vi "Signal Constructor.vi"(8 "error in (no error)":errorcluster, 11 "Signal Settings":T1) -> (0 "error out":errorcluster, 3 "IO Class.lvclass":refnum<class "Signal.lvclass">)   [LabVIEW 2025, in "Signal.lvclass"]
uses:
  Signal.lvclass
  Signal Settings.ctl
  Configuration.ctl
  VI/VI/Error Codes.ctl
  Digital Indicator/Digital Indicator.lvclass
  C:/Projects/VeriStand-FPGA-Generation-Wizard/Source/Classes/Signal/Signal/Signal.lvclass
  Digital Control/Digital Control.lvclass
  Analog Indicator/Analog Indicator.lvclass
  Analog Control/Analog Control.lvclass
  FPGA Addon Input/FPGA Addon Input.lvclass
  FPGA Addon Output/FPGA Addon Output.lvclass
  Quadrature Encoder Input/Quadrature Encoder Input.lvclass
  Wheel Speed Sensor/Wheel Speed Sensor.lvclass
  Signal.lvclass/Signal.ctl
  EST Digital Event/Digital Event.lvclass
  EST Output/EST Output.lvclass
  EST Knock Sensor/Knock Sensor.lvclass
  VI/VI/VI.lvclass
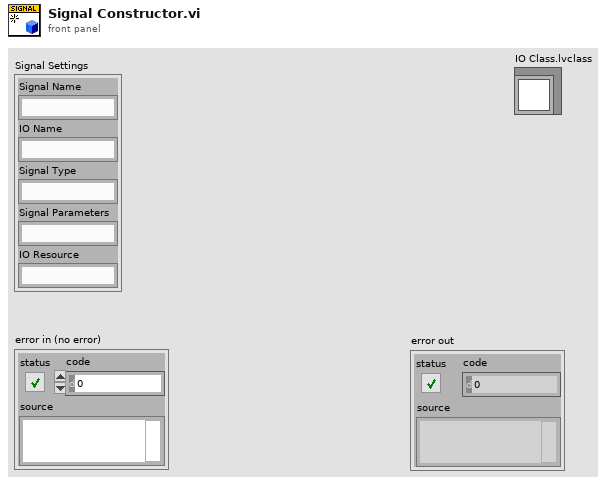
[diagram p1: front panel]
types:
  T1 = typedef "Signal.lvclass/Signal Settings.ctl" = cluster{"Signal Name":string, "IO Name":string, "Signal Type":string, "Signal Parameters":string, "IO Resource":string}
  T2 = typedef "VI.lvclass/Error Codes.ctl" = enum16{"Signal Unsupported", "Module Unsupported", "Parameter Unsupported", "Signal Code Gen Error", "Module Code Gen Error", "Cleanup Code Error", "Signal Direction Mismatch", "Signal Type Mismatch", "Module Channel Number Mismatch", "Minimum Channels Mismatch"}
  T3 = typedef "Signal.lvclass/Configuration.ctl" = cluster{"Classification":string, "Direction":string, "Type":string}
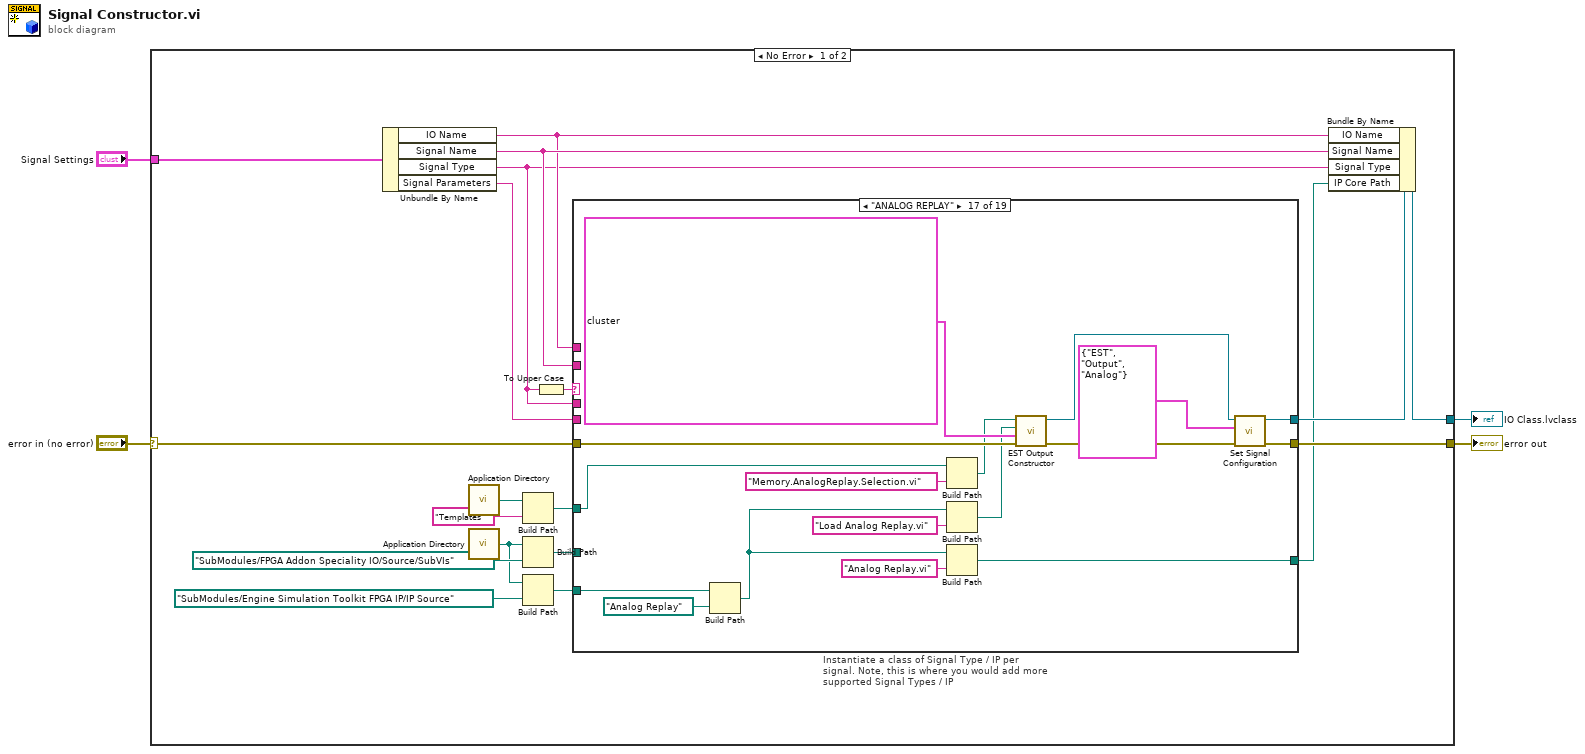
[diagram p0: block diagram]
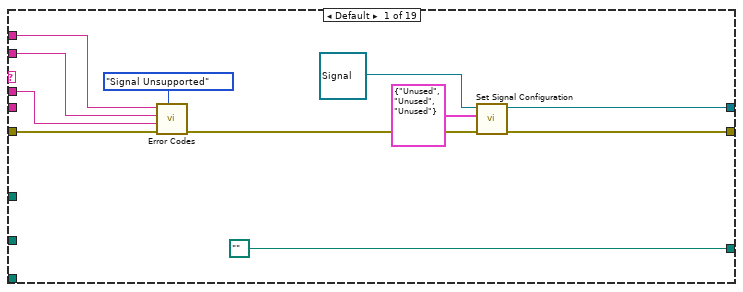
[diagram p2: hidden frame]
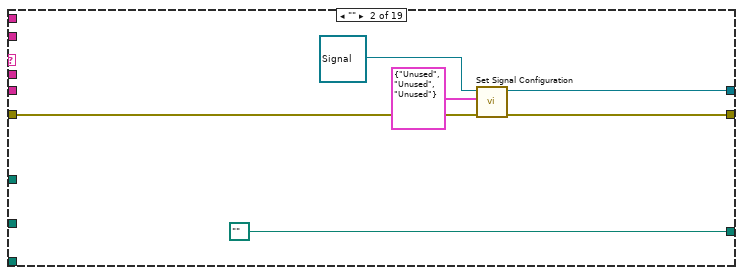
[diagram p3: hidden frame]
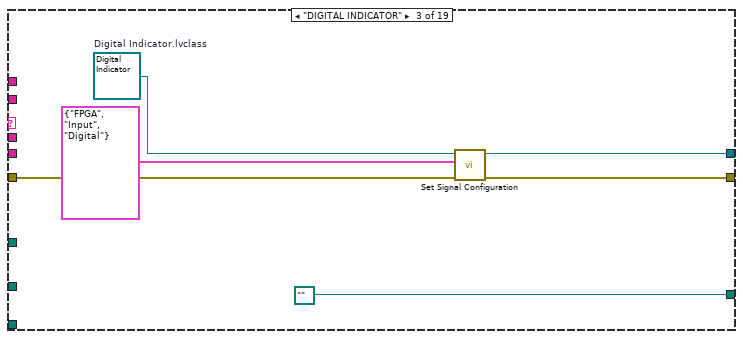
[diagram p4: hidden frame]
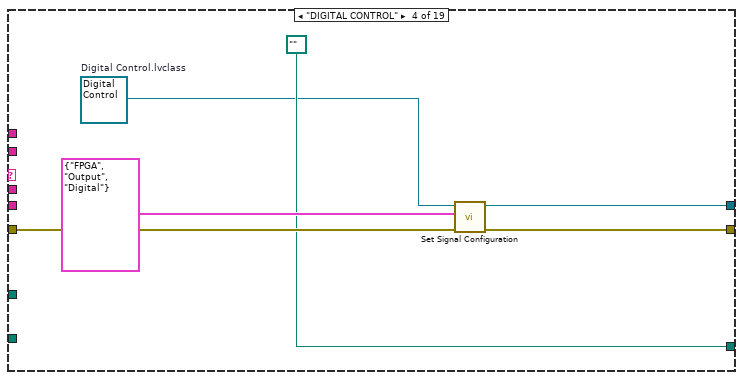
[diagram p5: hidden frame]
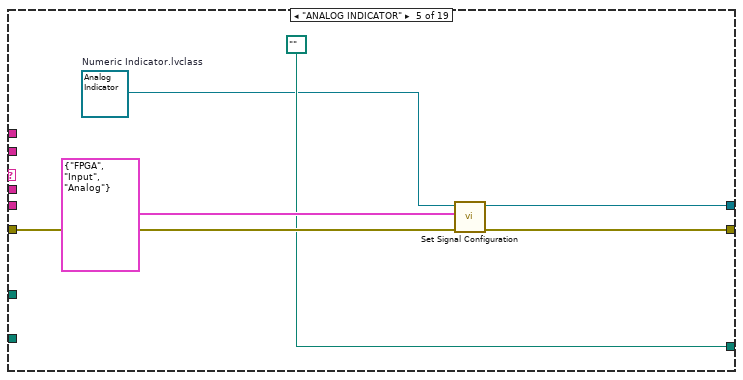
[diagram p6: hidden frame]
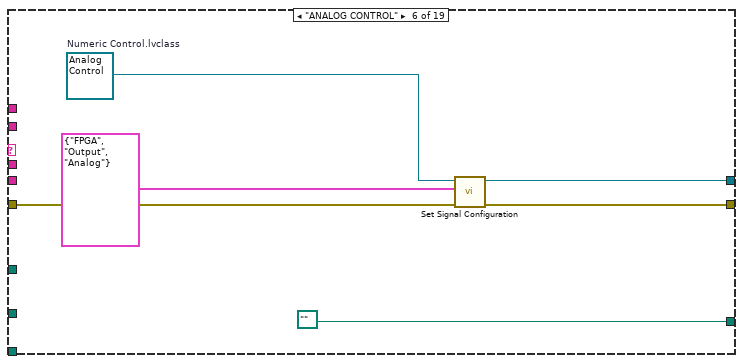
[diagram p7: hidden frame]
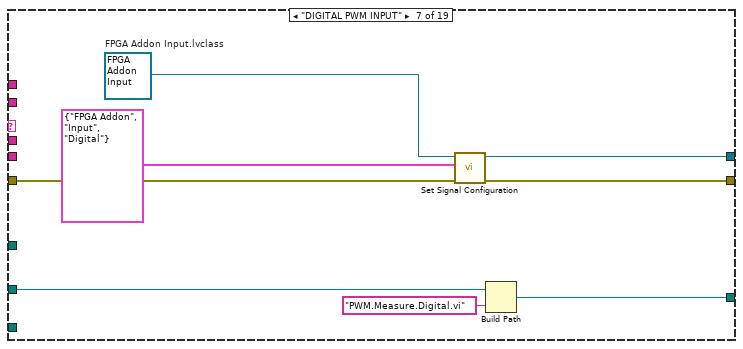
[diagram p8: hidden frame]
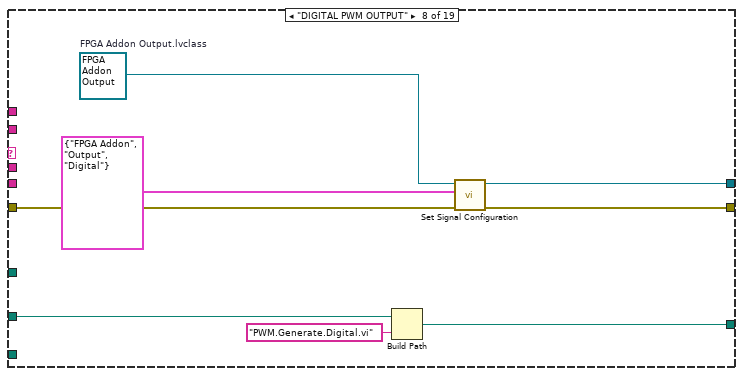
[diagram p9: hidden frame]
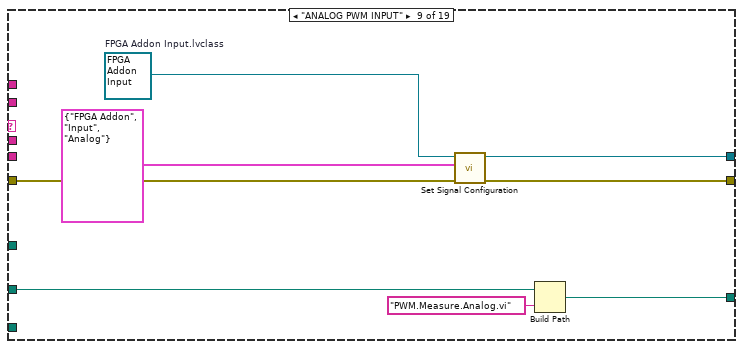
[diagram p10: hidden frame]
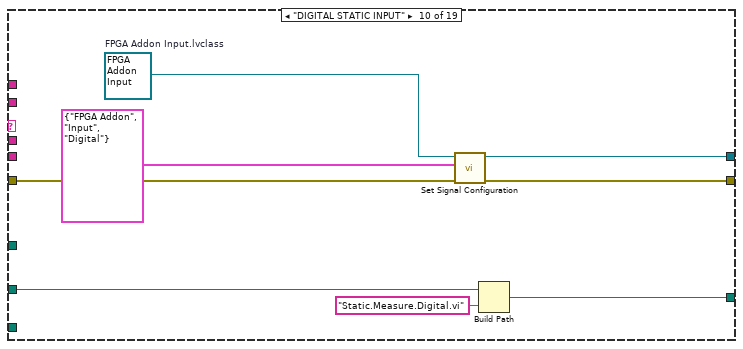
[diagram p11: hidden frame]
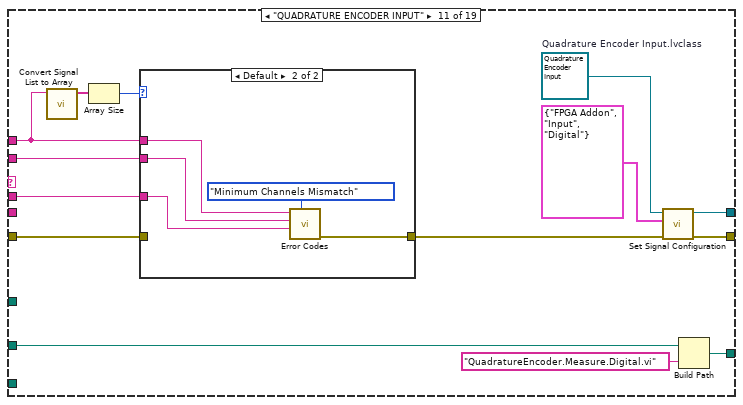
[diagram p12: hidden frame]
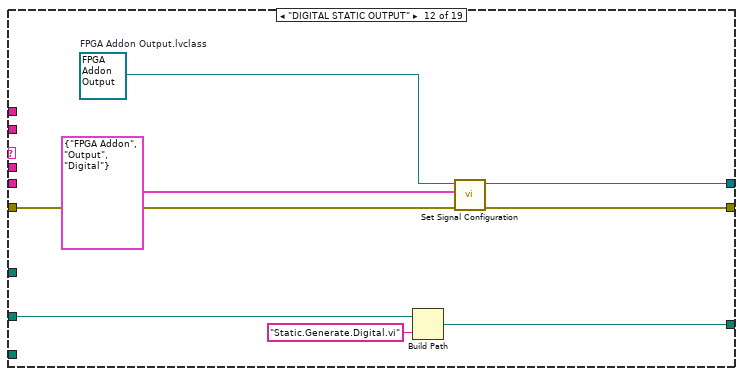
[diagram p14: hidden frame]
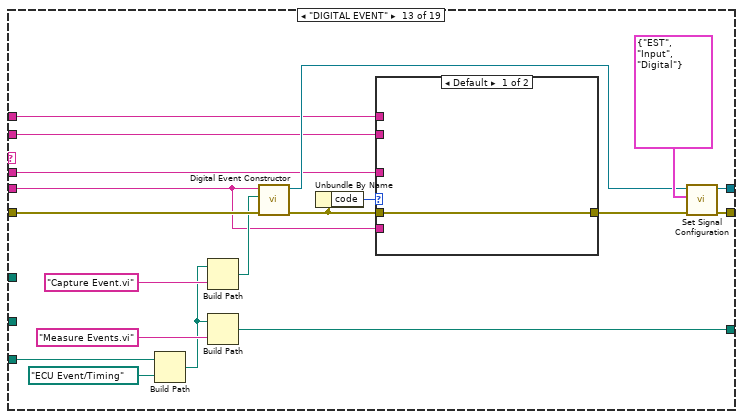
[diagram p15: hidden frame]
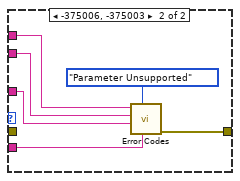
[diagram p16: hidden frame]
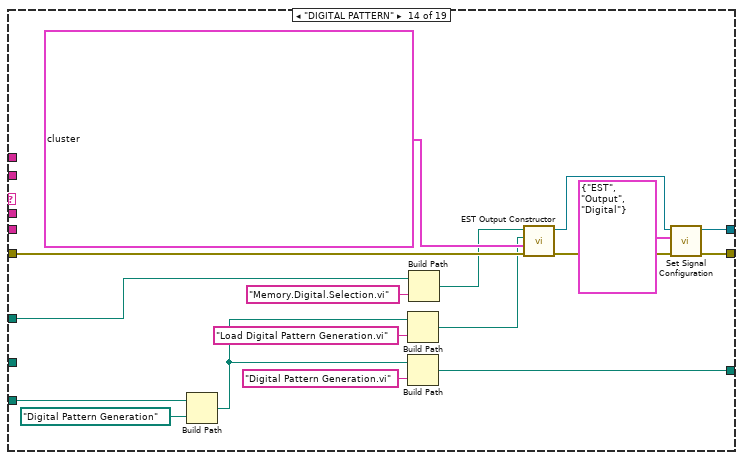
[diagram p17: hidden frame]
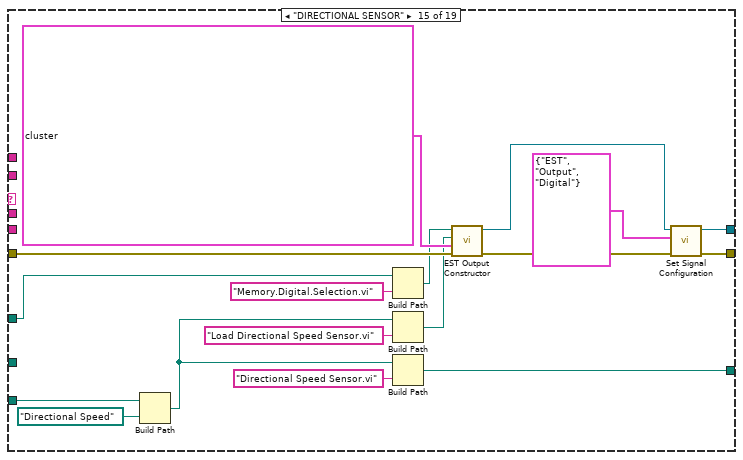
[diagram p18: hidden frame]
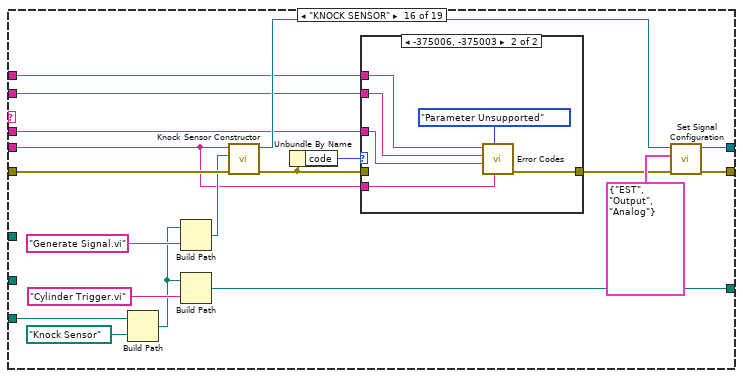
[diagram p19: hidden frame]
diagram:
  n1 = case shown="No Error" "error in (no error)" {
    selector: "error in (no error)" -> [w5 w257]
    tunnel: "Signal Settings" -> [w23 _]
    tunnel: [w21 w257] -> w3
    tunnel: [w20 refnum<class "Signal.lvclass"> refnum ("IO Class out")] -> w2
    frame No Error {
      n2 = Unbundle By Name(w23) -> ("IO Name"=w7:string, "Signal Name"=w8:string, "Signal Type"=w6:string, "Signal Parameters"=w19:string)
      n3 = call <vilib>:"Application Directory.vi"() -> ("Application Directory"=w11:path)
      n4 = call <vilib>:"Application Directory.vi"() -> ("Application Directory"=w9:path)
      n5 = Build Path(base path=w11, name or relative path="Templates") -> (appended path=w10:path)
      n6 = Build Path(base path=w9, name or relative path=path "SubModules/FPGA Addon Speciality IO/Source/SubVIs" ("path")) -> (appended path=w14:path)
      n7 = Build Path(base path=w9, name or relative path=path "SubModules/Engine Simulation Toolkit FPGA IP/IP Source" ("path")) -> (appended path=w13:path)
      n8 = To Upper Case(1:w6) -> (0:w22:string)
      n9 = case "Instantiate a class of Signal Type / IP per signal. Note, this is where you would add more supported Signal Types / IP" shown="\"ANALOG REPLAY\"" w22 {
        tunnel: w5 -> [w29 w35 w46 w52 w58 w64 w71 w80 w87 w95 w102 w124 w140 w164 w181 w200 w224 w235 w240]
        tunnel: [w33 w39 w45 w51 w57 w63 w70 w79 w86 w94 w110 w123 w143 w167 w184 w203 w227 w234 w249] -> w21
        tunnel: [w31 w37 w43 w49 w55 w61 w68 w77 w84 w92 w108 w121 w141 w165 w182 w201 w225 w232 w247] -> w18
        tunnel: w19 -> [_ _ _ _ _ _ _ _ _ _ _ _ w126 _ _ w185 _ _ _]
        tunnel: [path "" path "" path "" path "" path "" path "" w65 w73 w82 w89 w105 w117 w135 w155 w168 w195 w211 w228 w244] -> w17
        tunnel: w14 -> [_ _ _ _ _ _ w66 w74 w81 w90 w106 w118 _ _ _ _ _ w230 w246]
        tunnel: w13 -> [_ _ _ _ _ _ _ _ _ _ _ _ w138 w156 w171 w196 w215 _ _]
        tunnel: w10 -> [_ _ _ _ _ _ _ _ _ _ _ _ _ w153 w176 _ w214 _ _]
        tunnel: w8 -> [w27 _ _ _ _ _ _ _ _ _ w98 _ w127 _ _ w189 _ _ w237]
        tunnel: w7 -> [w26 _ _ _ _ _ _ _ _ _ w99 _ w128 _ _ w190 _ _ w236]
        tunnel: w6 -> [w24 _ _ _ _ _ _ _ _ _ w97 _ w125 _ _ w186 _ _ w238]
        frame Default {
          n10 = call "Error Codes.vi"("Error"=Error_Codes."Signal Unsupported", "error in (no error)"=w29, "Signal Type"=w24, "Module/Signal Name"=w27, "Module/Signal Resource"=w26) -> ("error out"=w28:errorcluster)  [unwired: 6 in]
          n11 = call "Set Signal Configuration.vi"("error in (no error)"=w28, "Configuration"=T3 {"Classification"="Unused", "Direction"="Unused", "Type"="Unused"}, "IO Class in"=refnum<class "Signal.lvclass"> refnum ("IO Class.lvclass")) -> ("error out"=w33:errorcluster, "IO Class out"=w31:refnum<class "Signal.lvclass">)  [unwired: 7 in]
        }
        frame "" {
          n12 = call "Set Signal Configuration.vi"("error in (no error)"=w35, "Configuration"=T3 {"Classification"="Unused", "Direction"="Unused", "Type"="Unused"}, "IO Class in"=refnum<class "Signal.lvclass"> refnum ("IO Class.lvclass")) -> ("error out"=w39:errorcluster, "IO Class out"=w37:refnum<class "Signal.lvclass">)  [unwired: 7 in]
        }
        frame "DIGITAL INDICATOR" {
          w41 = refnum<class "Digital Indicator.lvclass"> refnum  # Digital Indicator.lvclass
          n13 = call "Set Signal Configuration.vi"("error in (no error)"=w46, "Configuration"=T3 {"Classification"="FPGA", "Direction"="Input", "Type"="Digital"}, "IO Class in"=w41) -> ("error out"=w45:errorcluster, "IO Class out"=w43:refnum<class "Digital Indicator.lvclass">)  [unwired: 7 in]
        }
        frame "DIGITAL CONTROL" {
          w47 = refnum<class "Digital Control.lvclass"> refnum  # Digital Control.lvclass
          n14 = call "Set Signal Configuration.vi"("error in (no error)"=w52, "Configuration"=T3 {"Classification"="FPGA", "Direction"="Output", "Type"="Digital"}, "IO Class in"=w47) -> ("error out"=w51:errorcluster, "IO Class out"=w49:refnum<class "Digital Control.lvclass">)  [unwired: 7 in]
        }
        frame "ANALOG INDICATOR" {
          w53 = refnum<class "Analog Indicator.lvclass"> refnum  # Numeric Indicator.lvclass
          n15 = call "Set Signal Configuration.vi"("error in (no error)"=w58, "Configuration"=T3 {"Classification"="FPGA", "Direction"="Input", "Type"="Analog"}, "IO Class in"=w53) -> ("error out"=w57:errorcluster, "IO Class out"=w55:refnum<class "Analog Indicator.lvclass">)  [unwired: 7 in]
        }
        frame "ANALOG CONTROL" {
          w59 = refnum<class "Analog Control.lvclass"> refnum  # Numeric Control.lvclass
          n16 = call "Set Signal Configuration.vi"("error in (no error)"=w64, "Configuration"=T3 {"Classification"="FPGA", "Direction"="Output", "Type"="Analog"}, "IO Class in"=w59) -> ("error out"=w63:errorcluster, "IO Class out"=w61:refnum<class "Analog Control.lvclass">)  [unwired: 7 in]
        }
        frame "DIGITAL PWM INPUT" {
          w72 = refnum<class "FPGA Addon Input.lvclass"> refnum  # FPGA Addon Input.lvclass
          n17 = call "Set Signal Configuration.vi"("error in (no error)"=w71, "Configuration"=T3 {"Classification"="FPGA Addon", "Direction"="Input", "Type"="Digital"}, "IO Class in"=w72) -> ("error out"=w70:errorcluster, "IO Class out"=w68:refnum<class "FPGA Addon Input.lvclass">)  [unwired: 7 in]
          n18 = Build Path(base path=w66, name or relative path="PWM.Measure.Digital.vi") -> (appended path=w65:path)
        }
        frame "DIGITAL PWM OUTPUT" {
          w76 = refnum<class "FPGA Addon Output.lvclass"> refnum  # FPGA Addon Output.lvclass
          n19 = Build Path(base path=w74, name or relative path="PWM.Generate.Digital.vi") -> (appended path=w73:path)
          n20 = call "Set Signal Configuration.vi"("error in (no error)"=w80, "Configuration"=T3 {"Classification"="FPGA Addon", "Direction"="Output", "Type"="Digital"}, "IO Class in"=w76) -> ("error out"=w79:errorcluster, "IO Class out"=w77:refnum<class "FPGA Addon Output.lvclass">)  [unwired: 7 in]
        }
        frame "ANALOG PWM INPUT" {
          w88 = refnum<class "FPGA Addon Input.lvclass"> refnum  # FPGA Addon Input.lvclass
          n21 = call "Set Signal Configuration.vi"("error in (no error)"=w87, "Configuration"=T3 {"Classification"="FPGA Addon", "Direction"="Input", "Type"="Analog"}, "IO Class in"=w88) -> ("error out"=w86:errorcluster, "IO Class out"=w84:refnum<class "FPGA Addon Input.lvclass">)  [unwired: 7 in]
          n22 = Build Path(base path=w81, name or relative path="PWM.Measure.Analog.vi") -> (appended path=w82:path)
        }
        frame "DIGITAL STATIC INPUT" {
          w96 = refnum<class "FPGA Addon Input.lvclass"> refnum  # FPGA Addon Input.lvclass
          n23 = call "Set Signal Configuration.vi"("error in (no error)"=w95, "Configuration"=T3 {"Classification"="FPGA Addon", "Direction"="Input", "Type"="Digital"}, "IO Class in"=w96) -> ("error out"=w94:errorcluster, "IO Class out"=w92:refnum<class "FPGA Addon Input.lvclass">)  [unwired: 7 in]
          n24 = Build Path(base path=w90, name or relative path="Static.Measure.Digital.vi") -> (appended path=w89:path)
        }
        frame "QUADRATURE ENCODER INPUT" {
          w104 = refnum<class "Quadrature Encoder Input.lvclass"> refnum  # Quadrature Encoder Input.lvclass
          n25 = call "Convert Signal List to Array.vi"("Signal List"=w99) -> ("Signal List"=w103:string[])  [unwired: 10 in]
          n26 = Array Size(array=w103) -> (size(s)=w100:i32)
          n27 = case shown="Default" w100 {
            tunnel: w102 -> [w111 _]
            tunnel: [w111 w115] -> w101
            tunnel: w99 -> [_ w114]
            tunnel: w98 -> [_ w113]
            tunnel: w97 -> [_ w112]
            frame 3 {
            }
            frame Default {
              n28 = call "Error Codes.vi"("Error"=Error_Codes."Minimum Channels Mismatch", "Signal Type"=w112, "Module/Signal Name"=w113, "Module/Signal Resource"=w114) -> ("error out"=w115:errorcluster)  [unwired: 7 in]
            }
          }
          n29 = call "Set Signal Configuration.vi"("error in (no error)"=w101, "Configuration"=T3 {"Classification"="FPGA Addon", "Direction"="Input", "Type"="Digital"}, "IO Class in"=w104) -> ("error out"=w110:errorcluster, "IO Class out"=w108:refnum<class "Quadrature Encoder Input.lvclass">)  [unwired: 7 in]
          n30 = Build Path(base path=w106, name or relative path="QuadratureEncoder.Measure.Digital.vi") -> (appended path=w105:path)
        }
        frame "DIGITAL STATIC OUTPUT" {
          w120 = refnum<class "FPGA Addon Output.lvclass"> refnum  # FPGA Addon Output.lvclass
          n31 = Build Path(base path=w118, name or relative path="Static.Generate.Digital.vi") -> (appended path=w117:path)
          n32 = call "Set Signal Configuration.vi"("error in (no error)"=w124, "Configuration"=T3 {"Classification"="FPGA Addon", "Direction"="Output", "Type"="Digital"}, "IO Class in"=w120) -> ("error out"=w123:errorcluster, "IO Class out"=w121:refnum<class "FPGA Addon Output.lvclass">)  [unwired: 7 in]
        }
        frame "DIGITAL EVENT" {
          n33 = Build Path(base path=w138, name or relative path=path "ECU Event/Timing") -> (appended path=w133:path)
          n34 = Build Path(base path=w133, name or relative path="Capture Event.vi") -> (appended path=w132:path)
          n35 = Build Path(base path=w133, name or relative path="Measure Events.vi") -> (appended path=w135:path)
          n36 = call "Digital Event Constructor.vi"("error in (no error)"=w140, "Capture Path"=w132, "Signal Parameters"=w126) -> ("error out"=w130:errorcluster, "Digital Event.lvclass"=w139:refnum<class "Digital Event.lvclass">)  [unwired: 7 in]
          n37 = Unbundle By Name(w130) -> ("code"=w131:i32)
          n38 = case shown="Default" w131 {
            tunnel: w130 -> [w144 _]
            tunnel: [w144 w150] -> w129
            tunnel: w128 -> [_ w148]
            tunnel: w127 -> [_ w147]
            tunnel: w126 -> [_ w145]
            tunnel: w125 -> [_ w146]
            frame Default {
            }
            frame -375006, -375003 {
              n39 = call "Error Codes.vi"("Parameter"=w145, "Error"=Error_Codes."Parameter Unsupported", "Signal Type"=w146, "Module/Signal Name"=w147, "Module/Signal Resource"=w148) -> ("error out"=w150:errorcluster)  [unwired: 6 in]
            }
          }
          n40 = call "Set Signal Configuration.vi"("error in (no error)"=w129, "Configuration"=T3 {"Classification"="EST", "Direction"="Input", "Type"="Digital"}, "IO Class in"=w139) -> ("error out"=w143:errorcluster, "IO Class out"=w141:refnum<class "Digital Event.lvclass">)  [unwired: 7 in]
        }
        frame "DIGITAL PATTERN" {
          n41 = Build Path(base path=w156, name or relative path=path "Digital Pattern Generation") -> (appended path=w157:path)
          n42 = Build Path(base path=w157, name or relative path="Load Digital Pattern Generation.vi") -> (appended path=w154:path)
          n43 = Build Path(base path=w157, name or relative path="Digital Pattern Generation.vi") -> (appended path=w155:path)
          n44 = Build Path(base path=w153, name or relative path="Memory.Digital.Selection.vi") -> (appended path=w151:path)
          n45 = call "EST Output Constructor.vi"("error in (no error)"=w164, "Project Item"=cluster{"Name":string, "Value":variant}[] [{"Name"="FPGA.PersistentID", "Value"=variant(string "{CD7EB185-1A87-4E78-8C08-5D9A1491F439}")}, {"Name"="fullEmulation", "Value"=variant(bool TRUE)}, {"Name"="Memory Latency", "Value"=variant(u32 1)}, {"Name"="Multiple Clock Domains", "Value"=variant(bool FALSE)}, {"Name"="NI.LV.FPGA.CompileConfigString", "Value"=variant(string "Actual Number of Elements=1024;ReadArbs=2;WriteArbs=2;Implementation=2;DataType=100080000000000100094006000355313600010000000000000000;InitDataHash=;DRAM Selection=DramBank0;DRAM Max Outstanding Requests=64;DRAM Include Byte Enables=FALSE;DRAM Grant Time=50;Interface Configuration=Read A-Write B;Multiple Clock Domains=FALSE;Memory Latency=1")}, {"Name"="NI.LV.FPGA.MEMORY.ActualNumberOfElements", "Value"=variant(u32 1024)}, {"Name"="NI.LV.FPGA.MEMORY.DataWidth", "Value"=variant(u32 6)}, {"Name"="NI.LV.FPGA.MEMORY.DramIncludeByteEnables", "Value"=variant(bool FALSE)}, {"Name"="NI.LV.FPGA.MEMORY.DramMaxOutstandingRequests", "Value"=variant(i32 64)}, {"Name"="NI.LV.FPGA.MEMORY.DramSelection", "Value"=variant(string "DramBank0")}, {"Name"="NI.LV.FPGA.MEMORY.Init", "Value"=variant(bool FALSE)}, {"Name"="NI.LV.FPGA.MEMORY.InitData", "Value"=variant(string "")}, {"Name"="NI.LV.FPGA.MEMORY.InitVIPath", "Value"=variant(string "")}, {"Name"="NI.LV.FPGA.MEMORY.InterfaceAArbitration", "Value"=variant(u32 2)}, {"Name"="NI.LV.FPGA.MEMORY.InterfaceBArbitration", "Value"=variant(u32 2)}, {"Name"="NI.LV.FPGA.MEMORY.InterfaceConfig", "Value"=variant(u32 0)}, {"Name"="NI.LV.FPGA.MEMORY.RequestedNumberOfElements", "Value"=variant(u32 1024)}, {"Name"="NI.LV.FPGA.MEMORY.Type", "Value"=variant(u32 2)}, {"Name"="NI.LV.FPGA.ScriptConfigString", "Value"=variant(string "Actual Number of Elements=1024;ReadArbs=2;WriteArbs=2;Implementation=2;DataType=100080000000000100094006000355313600010000000000000000;InitDataHash=;DRAM Selection=DramBank0;DRAM Max Outstanding Requests=64;DRAM Include Byte Enables=FALSE;DRAM Grant Time=50;Interface Configuration=Read A-Write B;Multiple Clock Domains=FALSE;Memory Latency=1Persist Memory ValuesTRUE;")}, {"Name"="NI.LV.FPGA.Valid", "Value"=variant(bool TRUE)}, {"Name"="NI.LV.FPGA.Version", "Value"=variant(i32 10)}, {"Name"="Type Descriptor", "Value"=variant(string "100080000000000100094006000355313600010000000000000000")}] ("Array 2"), "Load Path"=w154, "Memory Template Path"=w151) -> ("error out"=w163:errorcluster, "EST Output.lvclass"=w162:refnum<class "EST Output.lvclass">)  [unwired: 6 in]
          n46 = call "Set Signal Configuration.vi"("error in (no error)"=w163, "Configuration"=T3 {"Classification"="EST", "Direction"="Output", "Type"="Digital"}, "IO Class in"=w162) -> ("error out"=w167:errorcluster, "IO Class out"=w165:refnum<class "EST Output.lvclass">)  [unwired: 7 in]
        }
        frame "DIRECTIONAL SENSOR" {
          n47 = Build Path(base path=w171, name or relative path=path "Directional Speed") -> (appended path=w170:path)
          n48 = Build Path(base path=w176, name or relative path="Memory.Digital.Selection.vi") -> (appended path=w175:path)
          n49 = Build Path(base path=w170, name or relative path="Load Directional Speed Sensor.vi") -> (appended path=w169:path)
          n50 = Build Path(base path=w170, name or relative path="Directional Speed Sensor.vi") -> (appended path=w168:path)
          n51 = call "EST Output Constructor.vi"("error in (no error)"=w181, "Project Item"=cluster{"Name":string, "Value":variant}[] [{"Name"="FPGA.PersistentID", "Value"=variant(string "{CD7EB185-1A87-4E78-8C08-5D9A1491F439}")}, {"Name"="fullEmulation", "Value"=variant(bool TRUE)}, {"Name"="Memory Latency", "Value"=variant(u32 1)}, {"Name"="Multiple Clock Domains", "Value"=variant(bool FALSE)}, {"Name"="NI.LV.FPGA.CompileConfigString", "Value"=variant(string "Actual Number of Elements=1024;ReadArbs=2;WriteArbs=2;Implementation=2;DataType=100080000000000100094006000355313600010000000000000000;InitDataHash=;DRAM Selection=DramBank0;DRAM Max Outstanding Requests=64;DRAM Include Byte Enables=FALSE;DRAM Grant Time=50;Interface Configuration=Read A-Write B;Multiple Clock Domains=FALSE;Memory Latency=1")}, {"Name"="NI.LV.FPGA.MEMORY.ActualNumberOfElements", "Value"=variant(u32 1024)}, {"Name"="NI.LV.FPGA.MEMORY.DataWidth", "Value"=variant(u32 6)}, {"Name"="NI.LV.FPGA.MEMORY.DramIncludeByteEnables", "Value"=variant(bool FALSE)}, {"Name"="NI.LV.FPGA.MEMORY.DramMaxOutstandingRequests", "Value"=variant(i32 64)}, {"Name"="NI.LV.FPGA.MEMORY.DramSelection", "Value"=variant(string "DramBank0")}, {"Name"="NI.LV.FPGA.MEMORY.Init", "Value"=variant(bool FALSE)}, {"Name"="NI.LV.FPGA.MEMORY.InitData", "Value"=variant(string "")}, {"Name"="NI.LV.FPGA.MEMORY.InitVIPath", "Value"=variant(string "")}, {"Name"="NI.LV.FPGA.MEMORY.InterfaceAArbitration", "Value"=variant(u32 2)}, {"Name"="NI.LV.FPGA.MEMORY.InterfaceBArbitration", "Value"=variant(u32 2)}, {"Name"="NI.LV.FPGA.MEMORY.InterfaceConfig", "Value"=variant(u32 0)}, {"Name"="NI.LV.FPGA.MEMORY.RequestedNumberOfElements", "Value"=variant(u32 1024)}, {"Name"="NI.LV.FPGA.MEMORY.Type", "Value"=variant(u32 2)}, {"Name"="NI.LV.FPGA.ScriptConfigString", "Value"=variant(string "Actual Number of Elements=1024;ReadArbs=2;WriteArbs=2;Implementation=2;DataType=100080000000000100094006000355313600010000000000000000;InitDataHash=;DRAM Selection=DramBank0;DRAM Max Outstanding Requests=64;DRAM Include Byte Enables=FALSE;DRAM Grant Time=50;Interface Configuration=Read A-Write B;Multiple Clock Domains=FALSE;Memory Latency=1Persist Memory ValuesTRUE;")}, {"Name"="NI.LV.FPGA.Valid", "Value"=variant(bool TRUE)}, {"Name"="NI.LV.FPGA.Version", "Value"=variant(i32 10)}, {"Name"="Type Descriptor", "Value"=variant(string "100080000000000100094006000355313600010000000000000000")}] ("Array 2"), "Load Path"=w169, "Memory Template Path"=w175) -> ("error out"=w180:errorcluster, "EST Output.lvclass"=w179:refnum<class "EST Output.lvclass">)  [unwired: 6 in]
          n52 = call "Set Signal Configuration.vi"("error in (no error)"=w180, "Configuration"=T3 {"Classification"="EST", "Direction"="Output", "Type"="Digital"}, "IO Class in"=w179) -> ("error out"=w184:errorcluster, "IO Class out"=w182:refnum<class "EST Output.lvclass">)  [unwired: 7 in]
        }
        frame "KNOCK SENSOR" {
          n53 = Build Path(base path=w196, name or relative path=path "Knock Sensor") -> (appended path=w193:path)
          n54 = Build Path(base path=w193, name or relative path="Generate Signal.vi") -> (appended path=w192:path)
          n55 = Build Path(base path=w193, name or relative path="Cylinder Trigger.vi") -> (appended path=w195:path)
          n56 = call "Knock Sensor Constructor.vi"("error in (no error)"=w200, "Generate Signal Path"=w192, "Signal Parameters"=w185) -> ("error out"=w188:errorcluster, "EST Knock Sensor.lvclass"=w199:refnum<class "Knock Sensor.lvclass">)  [unwired: 7 in]
          n57 = Unbundle By Name(w188) -> ("code"=w187:i32)
          n58 = case shown="-375006, -375003" w187 {
            tunnel: w188 -> [w204 _]
            tunnel: [w204 w210] -> w191
            tunnel: w190 -> [_ w208]
            tunnel: w189 -> [_ w207]
            tunnel: w186 -> [_ w206]
            tunnel: w185 -> [_ w205]
            frame Default {
            }
            frame -375006, -375003 {
              n59 = call "Error Codes.vi"("Parameter"=w205, "Error"=Error_Codes."Parameter Unsupported", "Signal Type"=w206, "Module/Signal Name"=w207, "Module/Signal Resource"=w208) -> ("error out"=w210:errorcluster)  [unwired: 6 in]
            }
          }
          n60 = call "Set Signal Configuration.vi"("error in (no error)"=w191, "Configuration"=T3 {"Classification"="EST", "Direction"="Output", "Type"="Analog"}, "IO Class in"=w199) -> ("error out"=w203:errorcluster, "IO Class out"=w201:refnum<class "Knock Sensor.lvclass">)  [unwired: 7 in]
        }
        frame "ANALOG REPLAY" {
          n61 = Build Path(base path=w215, name or relative path=path "Analog Replay") -> (appended path=w216:path)
          n62 = Build Path(base path=w214, name or relative path="Memory.AnalogReplay.Selection.vi") -> (appended path=w212:path)
          n63 = Build Path(base path=w216, name or relative path="Load Analog Replay.vi") -> (appended path=w213:path)
          n64 = Build Path(base path=w216, name or relative path="Analog Replay.vi") -> (appended path=w211:path)
          n65 = call "EST Output Constructor.vi"("error in (no error)"=w224, "Project Item"=cluster{"Name":string, "Value":variant}[] [{"Name"="FPGA.PersistentID", "Value"=variant(string "{CD7EB185-1A87-4E78-8C08-5D9A1491F439}")}, {"Name"="fullEmulation", "Value"=variant(bool TRUE)}, {"Name"="Memory Latency", "Value"=variant(u32 1)}, {"Name"="Multiple Clock Domains", "Value"=variant(bool FALSE)}, {"Name"="NI.LV.FPGA.CompileConfigString", "Value"=variant(string "Actual Number of Elements=16384;ReadArbs=2;WriteArbs=2;Implementation=2;DataType=100080000000000100094002000349313600010000000000000000;InitDataHash=;DRAM Selection=DramBank0;DRAM Max Outstanding Requests=64;DRAM Include Byte Enables=FALSE;DRAM Grant Time=50;Interface Configuration=Read A-Write B;Multiple Clock Domains=FALSE;Memory Latency=1")}, {"Name"="NI.LV.FPGA.MEMORY.ActualNumberOfElements", "Value"=variant(u32 16384)}, {"Name"="NI.LV.FPGA.MEMORY.DataWidth", "Value"=variant(u32 2)}, {"Name"="NI.LV.FPGA.MEMORY.DramIncludeByteEnables", "Value"=variant(bool FALSE)}, {"Name"="NI.LV.FPGA.MEMORY.DramMaxOutstandingRequests", "Value"=variant(i32 64)}, {"Name"="NI.LV.FPGA.MEMORY.DramSelection", "Value"=variant(string "DramBank0")}, {"Name"="NI.LV.FPGA.MEMORY.Init", "Value"=variant(bool FALSE)}, {"Name"="NI.LV.FPGA.MEMORY.InitData", "Value"=variant(string "")}, {"Name"="NI.LV.FPGA.MEMORY.InitVIPath", "Value"=variant(string "")}, {"Name"="NI.LV.FPGA.MEMORY.InterfaceAArbitration", "Value"=variant(u32 2)}, {"Name"="NI.LV.FPGA.MEMORY.InterfaceBArbitration", "Value"=variant(u32 2)}, {"Name"="NI.LV.FPGA.MEMORY.InterfaceConfig", "Value"=variant(u32 0)}, {"Name"="NI.LV.FPGA.MEMORY.RequestedNumberOfElements", "Value"=variant(u32 16384)}, {"Name"="NI.LV.FPGA.MEMORY.Type", "Value"=variant(u32 2)}, {"Name"="NI.LV.FPGA.ScriptConfigString", "Value"=variant(string "Actual Number of Elements=16384;ReadArbs=2;WriteArbs=2;Implementation=2;DataType=100080000000000100094002000349313600010000000000000000;InitDataHash=;DRAM Selection=DramBank0;DRAM Max Outstanding Requests=64;DRAM Include Byte Enables=FALSE;DRAM Grant Time=50;Interface Configuration=Read A-Write B;Multiple Clock Domains=FALSE;Memory Latency=1Persist Memory ValuesTRUE;")}, {"Name"="NI.LV.FPGA.Valid", "Value"=variant(bool TRUE)}, {"Name"="NI.LV.FPGA.Version", "Value"=variant(i32 10)}, {"Name"="Type Descriptor", "Value"=variant(string "100080000000000100094002000349313600010000000000000000")}] ("Array 2"), "Load Path"=w213, "Memory Template Path"=w212) -> ("error out"=w223:errorcluster, "EST Output.lvclass"=w222:refnum<class "EST Output.lvclass">)  [unwired: 6 in]
          n66 = call "Set Signal Configuration.vi"("error in (no error)"=w223, "Configuration"=T3 {"Classification"="EST", "Direction"="Output", "Type"="Analog"}, "IO Class in"=w222) -> ("error out"=w227:errorcluster, "IO Class out"=w225:refnum<class "EST Output.lvclass">)  [unwired: 7 in]
        }
        frame "SINE OUTPUT" {
          w231 = refnum<class "FPGA Addon Output.lvclass"> refnum  # FPGA Addon Output.lvclass
          n67 = Build Path(base path=w230, name or relative path="Sine.Generate.vi") -> (appended path=w228:path)
          n68 = call "Set Signal Configuration.vi"("error in (no error)"=w235, "Configuration"=T3 {"Classification"="FPGA Addon", "Direction"="Output", "Type"="Analog"}, "IO Class in"=w231) -> ("error out"=w234:errorcluster, "IO Class out"=w232:refnum<class "FPGA Addon Output.lvclass">)  [unwired: 7 in]
        }
        frame "WHEEL SPEED SENSOR" {
          w243 = refnum<class "Wheel Speed Sensor.lvclass"> refnum  # Wheel Speed Sensor.lvclass
          n69 = call "Convert Signal List to Array.vi"("Signal List"=w236) -> ("Signal List"=w242:string[])  [unwired: 10 in]
          n70 = Array Size(array=w242) -> (size(s)=w241:i32)
          n71 = case shown="Default" w241 {
            tunnel: w240 -> [w250 _]
            tunnel: [w250 w254] -> w239
            tunnel: w236 -> [_ w253]
            tunnel: w237 -> [_ w252]
            tunnel: w238 -> [_ w251]
            frame 2 {
            }
            frame Default {
              n72 = call "Error Codes.vi"("Error"=Error_Codes."Minimum Channels Mismatch", "Signal Type"=w251, "Module/Signal Name"=w252, "Module/Signal Resource"=w253) -> ("error out"=w254:errorcluster)  [unwired: 7 in]
            }
          }
          n73 = Build Path(base path=w246, name or relative path="WSS.Generate.Digital.vi") -> (appended path=w244:path)
          n74 = call "Set Signal Configuration.vi"("error in (no error)"=w239, "Configuration"=T3 {"Classification"="FPGA Addon", "Direction"="Output", "Type"="Digital"}, "IO Class in"=w243) -> ("error out"=w249:errorcluster, "IO Class out"=w247:refnum<class "Wheel Speed Sensor.lvclass">)  [unwired: 7 in]
        }
      }
      n75 = Bundle By Name(cluster=w18, "IO Name"=w7, "Signal Name"=w8, "Signal Type"=w6, "IP Core Path"=w17) -> (w20:refnum<class "Signal.lvclass">)
    }
    frame Error {
    }
  }
  "error out" <- w3
  "IO Class.lvclass" <- w2
